vi "Solve Band Linear Equations (single right hand).vi"(8 "Known Vector":dbl[](array[numeric]) format="%.2f", 9 "# of super-diagonal":i32, 10 "# of sub-diagonal":i32, 11 "Banded Matrix":dbl[][](array[numeric]) format="%.2f") -> (0 "error":i32, 3 "Solution Vector":dbl[](array[numeric]) format="%.2f")   [LabVIEW 2014, in "NI_AALPro.lvlib"]
doc: "Computes the solution to the system of linear equations AX=Y with a band coefficient matrix A and single or multiple right-hand sides Y."
uses:
  NI_AALPro.lvlib
  lvanlys.dll
panel:
  out "Band Storage":string[][](table)=[["*", "a01", "a12", "a23", "a34", "a45"], ["a00", "a11", "a22", "a33", "a44", "a55"], ["a10", "a21", "a32", "a43", "a54", "*"], ["a20", "a31", "a42", "a53", "*", "*"]]
  out "Banded Matrix with order=6, #sub-diagonal=2 and #super-diagonal=1":string[][](table)=[["a00", "a01", "0", "0", "0", "0"], ["a10", "a11", "a12", "0", "0", "0"], ["a20", "a21", "a22", "a23", "0", "0"], ["0", "a31", "a32", "a33", "a34", "0"], ["0", "0", "a42", "a43", "a44", "a45"], ["0", "0", "0", "a53", "a54", "a55"]]
  # "Solve Band Linear Equations"
  # "Must be in band storage"
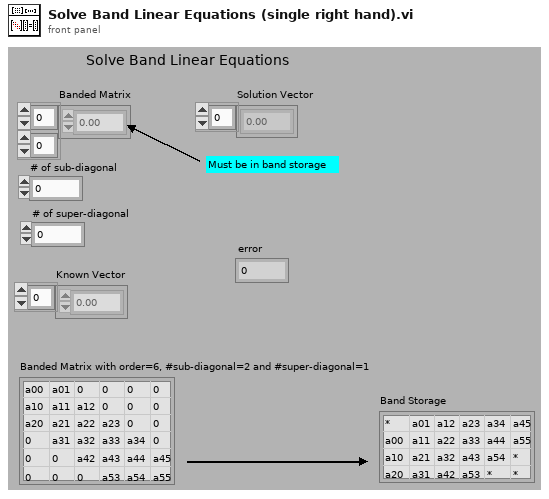
[diagram p1: front panel]
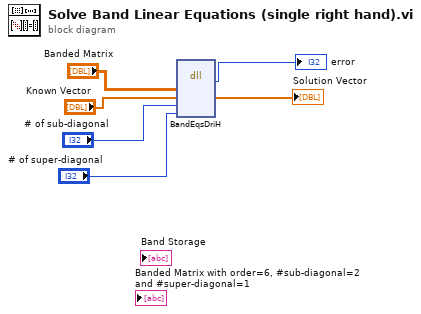
[diagram p0: block diagram]
diagram:
  n1 = dll-call lib="C:/Program Files (x86)/National Instruments/LabVIEW 2014/resource/lvanlys.*" fn="BandEqsDriH"("Banded Matrix"="Banded Matrix", "Known Vector"="Known Vector", "kl"="# of sub-diagonal", "ku"="# of super-diagonal") -> (→"error":i32, "Known Vector"=→"Solution Vector":dbl[])  [unwired: 6 in, 2 out]
